vi "Ustaw Gen Sygnal VI.vi"(10 "Ksztalt sygnalu":T1(ring)) -> (1 "generowany sygnal":waveform(dbl))   [LabVIEW 2015]
uses:
  <vilib>/measure/NI_MABase.lvlib
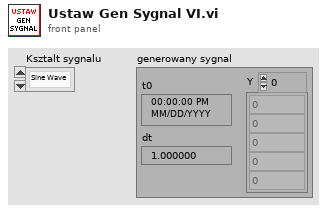
[diagram p1: front panel]
types:
  T1 = enum16{"Sine Wave", "Triangle Wave", "Square Wave", "Sawtooth Wave"}
  T2 = cluster{"Czestotliwosc probkowania":dbl, "Liczba probek":dbl}
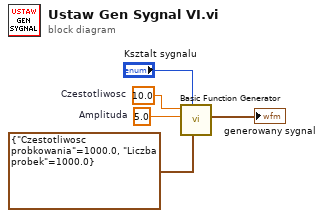
[diagram p0: block diagram]
diagram:
  w2 = 5.0  # Amplituda
  w3 = 10.0  # Czestotliwosc
  n1 = call <vilib>:"Basic Function Generator.vi"("sampling info"=T2 {"Czestotliwosc probkowania"=1000.0, "Liczba probek"=1000.0}, "signal type"="Ksztalt sygnalu", "amplitude"=w2, "frequency"=w3) -> ("signal out"=→"generowany sygnal":waveform(dbl))  [unwired: 5 in, 2 out]
